vi "Close SP.vi"(8 "error in (no error)":errorcluster, 11 "Auto UI in":refnum<class "Auto UI.lvclass">) -> (0 "error out":errorcluster, 3 "Auto UI out":refnum<class "Auto UI.lvclass">)   [LabVIEW 2023, in "GUI.lvlib" / "Auto UI.lvlib" / "Auto UI.lvclass"]
uses:
  Auto UI.lvclass
  Reused Code/Subpanels Actor/subpanels/subpanel/subpanel (abstract).lvclass
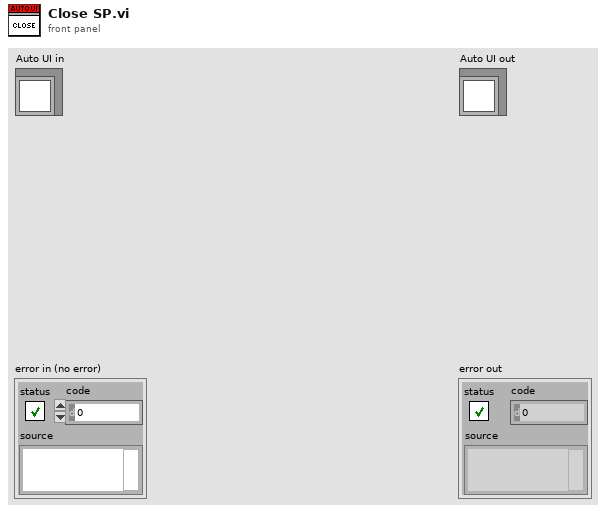
[diagram p1: front panel]
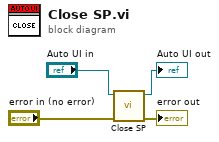
[diagram p0: block diagram]
diagram:
  n1 = call-parent "Close SP.vi"("error in (no error)"="error in (no error)", "subpanel (abstract) in"="Auto UI in") -> ("error out"=→"error out":errorcluster, "subpanel (abstract) out"=→"Auto UI out":refnum<class "Auto UI.lvclass">)  [unwired: 8 in]
